vi "Read XML_Parse RT modeCodes.vi"(8 "error in (no error)":errorcluster, 10 "RT in":T1, 11 "remoteTerminal in":refnum<k24>) -> (0 "error out":errorcluster, 2 "RT out":T1, 3 "remoteTerminal out":refnum<k24>)   [LabVIEW 2020, in "Ballard 1553 System Explorer.lvlib"]
uses:
  Ballard 1553 System Explorer.lvlib
  Ballard_RT.ctl
  Ballard_RT subAddress.ctl
  Ballard_RT direction.ctl
  Ballard_RT rtMode.ctl
  Ballard_RT modeCode.ctl
  C:/Users/Administrator/Desktop/GIT/Ballard-MIL-STD-1553-Custom-Device/Source/System Explorer/SubVIs/Parse XML Ballard/1.2/BTIXML_SerDes.dll
  1.2/BTIXML_SerDes.dll
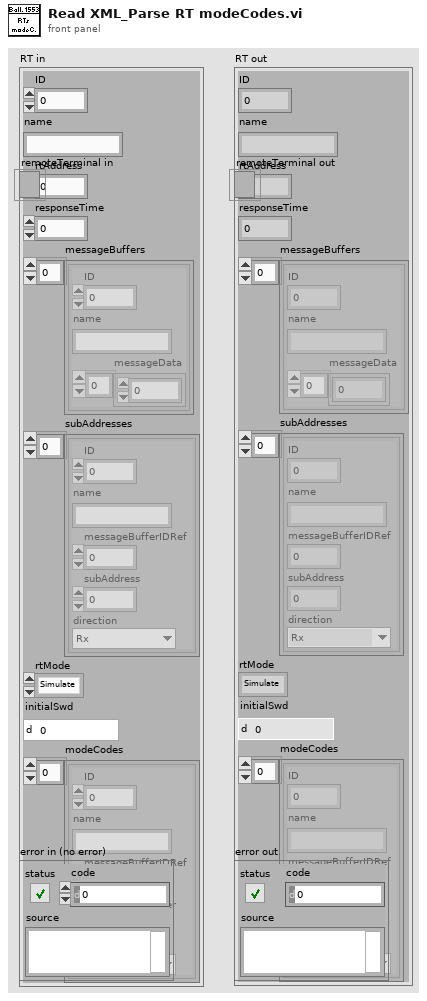
[diagram p1: front panel]
types:
  T1 = typedef "Ballard 1553 System Explorer.lvlib/Ballard_RT.ctl" = cluster{"ID":i32, "name":string, "rtAddress":i8, "responseTime":i32, "messageBuffers":cluster{"ID":i32, "name":string, "messageData":u16[]}[], "subAddresses":T2[], "rtMode":T4, "initialSwd":u16, "modeCodes":T5[]}
  T2 = typedef "Ballard 1553 System Explorer.lvlib/Ballard_RT subAddress.ctl" = cluster{"ID":i32, "name":string, "messageBufferIDRef":i32, "subAddress":i8, "direction":T3}
  T3 = typedef "Ballard 1553 System Explorer.lvlib/Ballard_RT direction.ctl" = enum16{"Tx", "Rx"}
  T4 = typedef "Ballard 1553 System Explorer.lvlib/Ballard_RT rtMode.ctl" = enum16{"Simulate", "Monitor", "Disable"}
  T5 = typedef "Ballard 1553 System Explorer.lvlib/Ballard_RT modeCode.ctl" = cluster{"ID":i32, "name":string, "messageBufferIDRef":i32, "modeCodeNumber":i8, "direction":T3}
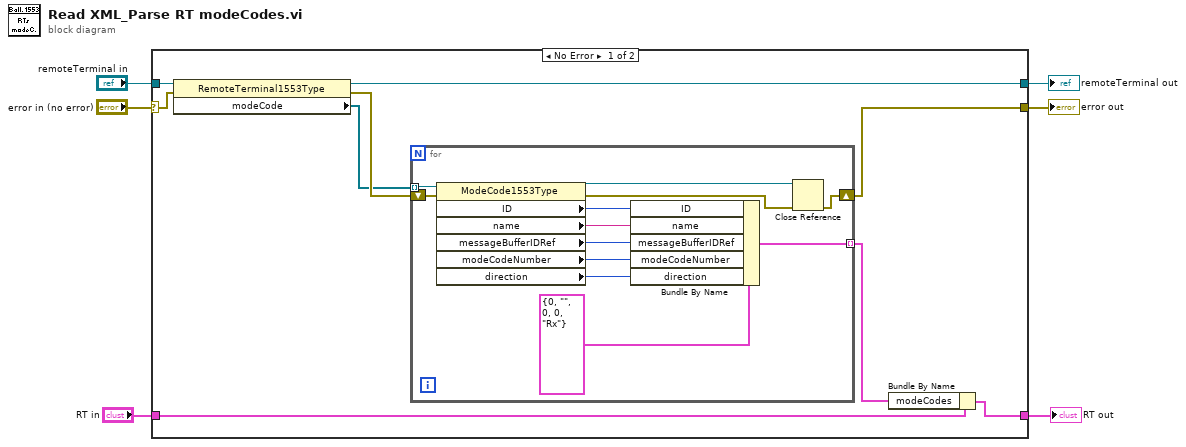
[diagram p0: block diagram]
diagram:
  n1 = case shown="No Error" "error in (no error)" {
    selector: "error in (no error)" -> [w8 w29]
    tunnel: [w15 w28] -> w6
    tunnel: "RT in" -> [w13 w28]
    tunnel: [w7 w29] -> w4
    tunnel: [w10 w30] -> w3
    tunnel: "remoteTerminal in" -> [w9 w30]
    frame No Error {
      n2 = property class="RemoteTerminal1553Type"(reference=w9, error in=w8) -> (reference out=w10:refnum<k24>, error out=w12:errorcluster, "modeCode"=w11:refnum<k24>[])
      n3 = for {
        tunnel: w11 -> [w27] mode=indexing
        tunnel: [w20] -> w14 mode=indexing
        shift-right: [w17] -> w7
        shift-left: w12 -> [w26]
        n4 = property class="ModeCode1553Type"(reference=w27, error in=w26) -> (reference out=w18:refnum<k24>, error out=w19:errorcluster, "ID"=w24:i32, "name"=w23:string, "messageBufferIDRef"=w22:i32, "modeCodeNumber"=w16:i8, "direction"=w21:i32)
        n5 = Bundle By Name(cluster=T5 {"ID"=0, "name"="", "messageBufferIDRef"=0, "modeCodeNumber"=0, "direction"=enum."Rx"} ("subAddress"), "ID"=w24, "name"=w23, "messageBufferIDRef"=w22, "modeCodeNumber"=w16, "direction"=w21) -> (w20:T5)
        n6 = Close Reference(reference=w18, error in (no error)=w19) -> (error out=w17:errorcluster)
      }
      n7 = Bundle By Name(cluster=w13, "modeCodes"=w14) -> (w15:T1)
    }
    frame Error {
    }
  }
  "RT out" <- w6
  "error out" <- w4
  "remoteTerminal out" <- w3
